vi "TagDB Multi-Thread Example.vi"() -> ()   [LabVIEW 2017]
uses:
  a657961d-6c69-443e-8a94-87e847e8afca.vi
  46a5d0b1-31a7-4634-b485-2dd57def936d.vi
  d2a29e7f-7a10-4ef4-95c2-af8e2a57b835.vi
  fda3db9f-a2b2-414c-9bd7-69cd5009c9b8.vi
  TagDB/_Support/DataAccess/data-Write.vi
  TagDB/_Support/Error/_[error50000]Invalid DB REF.vi
  TagDB/_Support/DataAccess/TagDB Ref to DVR.vi
  TagDB/_Support/DataAccess/_NameCacher.vi
  TagDB/_Support/Error/_[error50002]Invalid DataType.vi
  TagDB/_Support/URL/TRIM-BOTH-SPACE.vi
  TagDB/_Support/DataAccess/_datatypeChecker.vi
  <vilib>/Utility/Data Type/Get Type Information.vi
  TagDB/_Support/Error/_Build Error Cluster.vi
  TagDB/TagDB.lvlib
panel:
  out "version":string
  in  "stop":bool
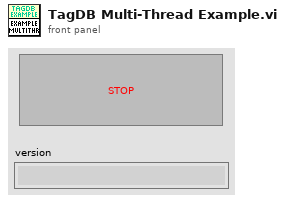
[diagram p1: front panel]
types:
  T1 = cluster{"number":i32, "boolean":bool, "abcdef":cluster{"number":i32, "boolean":bool}}
  T2 = typedef "TagDB.lvlib/TagDB.ctl" = refnum<k1>
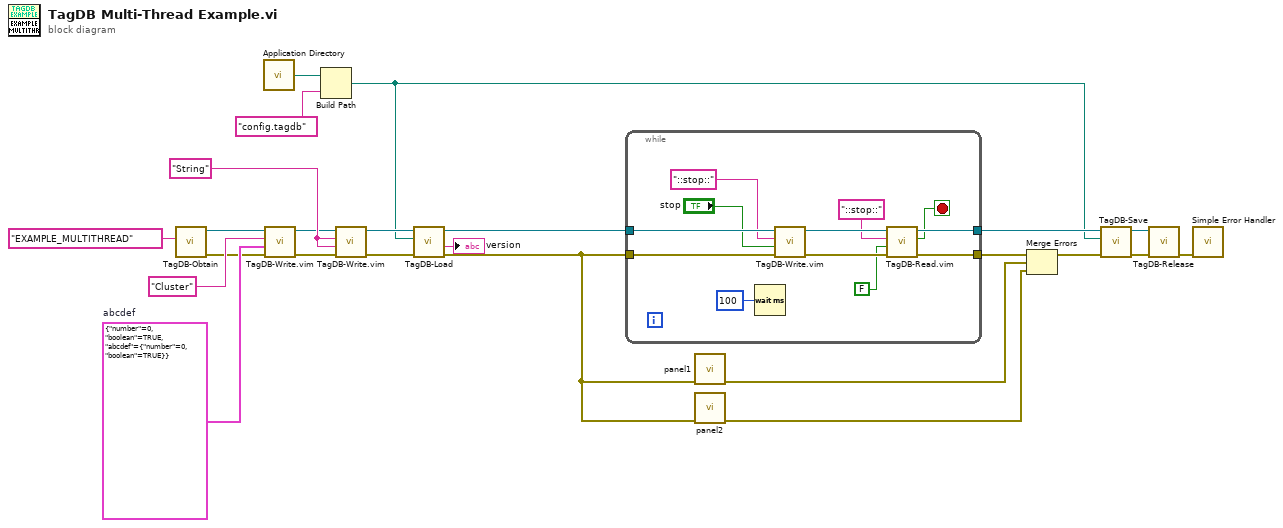
[diagram p0: block diagram]
diagram:
  w10 = T1 {"number"=0, "boolean"=TRUE, "abcdef"={"number"=0, "boolean"=TRUE}}  # abcdef
  w16 = "String" ("String")
  n1 = call "TagDB-Obtain.vi"("name (unnamed)"="EXAMPLE_MULTITHREAD") -> ("error out"=w5:errorcluster, "TagDB"=w6:T2)  [unwired: 4 in, 1 out]
  n2 = call <vilib>:"Application Directory.vi"() -> ("Application Directory"=w22:path)
  n3 = call "TagDB-Write.vim"("error in (no error)"=w5, "Value"=w10, "tag"="Cluster" ("name"), "TagDB"=w6) -> ("error out"=w12:errorcluster, "TagDB(dup)"=w13:T2)  [unwired: 5 in, 1 out]
  n4 = Build Path(base path=w22, name or relative path="config.tagdb") -> (appended path=w7:path)
  n5 = call "TagDB-Write.vim"("error in (no error)"=w12, "Value"=w16, "tag"=w16, "TagDB"=w13) -> ("error out"=w17:errorcluster, "TagDB(dup)"=w18:T2)  [unwired: 5 in, 1 out]
  n6 = call "TagDB-Load.vi"("error in (no error)"=w17, "file path(empty for default)"=w7, "DB Ref"=w18) -> ("error out"=w14:errorcluster, "version"=→"version":string, "DB Ref(dup)"=w15:T2)  [unwired: 6 in]
  n7 = while {
    tunnel: w15 -> [w34]
    tunnel: w14 -> [w35]
    tunnel: [w27] -> w2
    tunnel: [w30] -> w20
    stop <- w26 stop-if-true
    n8 = Wait (ms)(milliseconds to wait=u32 100) -> ()  [unwired: 1 out]
    n9 = call "TagDB-Write.vim"("error in (no error)"=w35, "Value"="stop", "tag"="::stop::" ("name"), "TagDB"=w34) -> ("error out"=w28:errorcluster, "TagDB(dup)"=w31:T2)  [unwired: 5 in, 1 out]
    n10 = call "TagDB-Read.vim"("error in (no error)"=w28, "Type(empty to read as variant)"=FALSE, "name"="::stop::", "TagDB"=w31) -> ("error out"=w27:errorcluster, "Value"=w26:bool, "TagDB(dup)"=w30:T2)  [unwired: 2 in, 3 out]
  }
  n11 = call "panel1.vi"("error in (no error)"=w14) -> ("error out"=w1:errorcluster)  [unwired: 10 in]
  n12 = call "panel2.vi"("error in (no error)"=w14) -> ("error out"=w23:errorcluster)  [unwired: 10 in]
  n13 = Merge Errors(w2, w1, w23) -> (w19:errorcluster)
  n14 = call "TagDB-Save.vi"("error in (no error)"=w19, "file path(empty for default)"=w7, "DB Ref"=w20) -> ("error out"=w8:errorcluster, "DB Ref(dup)"=w9:T2)  [unwired: 7 in]
  n15 = call "TagDB-Release.vi"("error in (no error)"=w8, "TagDB"=w9) -> ("error out"=w24:errorcluster)  [unwired: 9 in]
  n16 = call <vilib>:"Simple Error Handler.vi"("error in (no error)"=w24) -> ()  [unwired: 4 in, 5 out]
